vi "func.vi"() -> ()   [LabVIEW 2017]
panel:
  in  "?":bool
  out "Температура":dbl
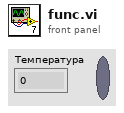
[diagram p1: front panel]
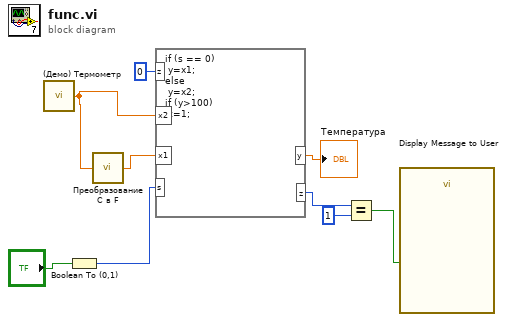
[diagram p0: block diagram]
diagram:
  n1 = call "(Демо) Термометр.vi"() -> ("Температура"=w5:dbl)  [unwired: 1 in]
  n2 = Boolean To (0,1)(Boolean="?") -> (0, 1=w7:i16)
  n3 = call "Преобразование C в F.vi"("Град C"=w5) -> ("Град F"=w6:dbl)
  n4 = formula code="if (s == 0)\n\ty=x1;\nelse\n\ty=x2;\nif (y>100)\n z=1;"("x1"=w6, "s"=w7, "x2"=w5, "z"=0 ("input variable")) -> ("y"=→"Температура":dbl, "z"=w3:i32)
  n5 = Equal?(x=w3, y=1) -> (x = y?=w1:bool)
  n6 = call "Display Message to User"("Enable"=w1) -> ()  [unwired: 9 in, 2 out]
